vi "byte_4_2bit.vi"(11 "BYTE":u8) -> (0 "6 7":u8, 1 "4 5":u8, 2 "2 3":u8, 3 "0 1":u8)   [LabVIEW 2016]
panel:
  # "一个字节每两位分开"
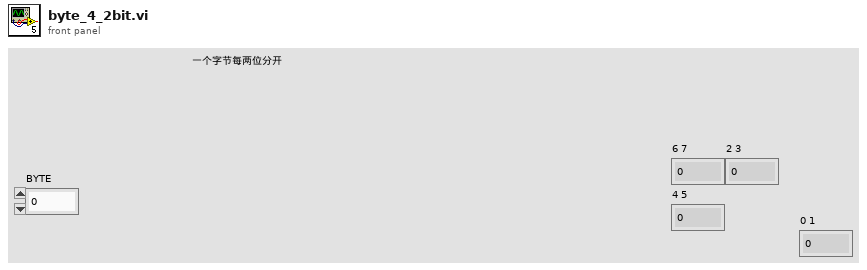
[diagram p1: front panel]
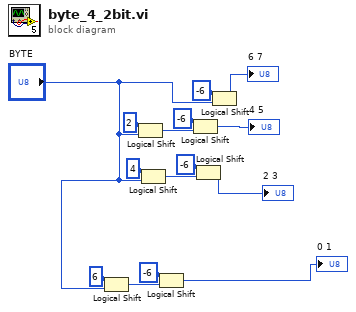
[diagram p0: block diagram]
diagram:
  n1 = Logical Shift(y=i16 6, x="BYTE") -> (x << y=w5:u8)
  n2 = Logical Shift(y=i16 2, x="BYTE") -> (x << y=w14:u8)
  n3 = Logical Shift(y=i16 4, x="BYTE") -> (x << y=w9:u8)
  n4 = Logical Shift(y=i16 -6, x=w5) -> (x << y=→"0 1":u8)
  n5 = Logical Shift(y=i16 -6, x=w14) -> (x << y=→"4 5":u8)
  n6 = Logical Shift(y=i16 -6, x=w9) -> (x << y=→"2 3":u8)
  n7 = Logical Shift(y=i16 -6, x="BYTE") -> (x << y=→"6 7":u8)
